vi "DriveFineAjust.vi"(8 "Fine Ajust F/B":dbl, 9 "Fine Ajust L/R":dbl, 10 "Right Side Normal":dbl, 11 "Left Side Normal":dbl) -> ()   [LabVIEW 2012]
uses:
  <vilib>/Rock Robotics/WPI/RobotDrive/WPI_RobotDriveGetSetRefNum.vi
  Max'sToolKit/ConvertVoltageToPercentVbs.vi
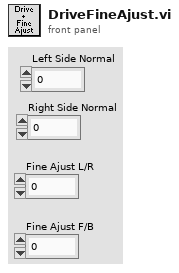
[diagram p1: front panel]
types:
  T1 = typedef "WPI_RobotDriveDevRef.ctl" = cluster{"DevStatus":errorcluster, "Motors[]":T2[], "Square Inputs":bool, "Max Output":dbl, "Isochronous":bool}
  T2 = typedef "WPI_MotorControlDeviceRef.ctl" = cluster{"DeviceStatus":errorcluster, "Type":enum16{"PWM", "CAN"}, "PWM":cluster{"Digital Module":T3, "PWM Channel":T4, "DeadBand":T5}, "CAN":cluster{"Device Number":u8, "Control Mode":T6, "Semaphore":T7, "Max Vout":dbl}, "Invert":bool, "TransformRef":T8, "InvTransformRef":T8}
  T3 = typedef "FPGA_TypedefDigitalModule.ctl" = enum16{"Digital Module 1", "Digital Module 2"}
  T4 = typedef "FPGA_DIOPWMChannel.ctl" = enum8{"PWM 1", "PWM 2", "PWM 3", "PWM 4", "PWM 5", "PWM 6", "PWM 7", "PWM 8", "PWM 9", "PWM 10", "Invalid"}
  T5 = typedef "WPI_PWMDeadband.ctl" = cluster{"Name":string, "maxPositivePwm":i32, "minPositivePwm":i32, "centerPwm":i32, "maxNegativePwm":i32, "minNegativePwm":i32, "angularRange":u16}
  T6 = typedef "WPI_CANJaguar_ControlMode.ctl" = enum8{"Percent VBus", "Current", "Speed", "Position", "Voltage"}
  T7 = typedef "Semaphore RefNum" = refnum<k1>
  T8 = typedef "WPI_PWMTransform_ConPane.ctl" = refnum<vi>
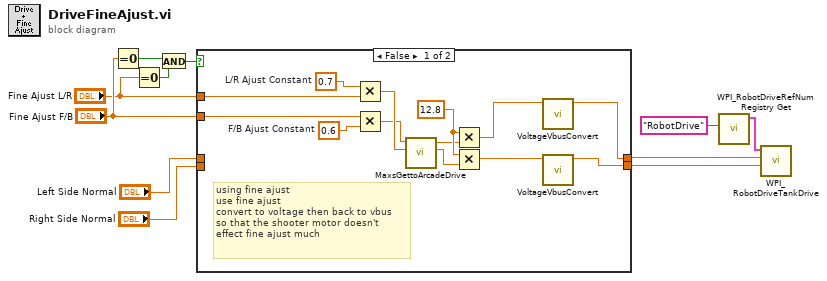
[diagram p0: block diagram]
diagram:
  n1 = Equal To 0?(x="Fine Ajust F/B") -> (x = 0?=w4:bool)
  n2 = Equal To 0?(x="Fine Ajust L/R") -> (x = 0?=w5:bool)
  n3 = And(x=w4, y=w5) -> (x .and. y?=w6:bool)
  n4 = case shown="False" w6 {
    tunnel: "Right Side Normal" -> [_ w25]
    tunnel: "Left Side Normal" -> [_ w26]
    tunnel: "Fine Ajust L/R" -> [w23 _]
    tunnel: "Fine Ajust F/B" -> [w21 _]
    tunnel: [w13 w26] -> w3
    tunnel: [w12 w25] -> w1
    frame False {
      w18 = 12.8
      w22 = 0.6  # F/B Ajust Constant
      w24 = 0.7  # L/R Ajust Constant
      # "using fine ajust\nuse fine ajust\nconvert to voltage then back to vbus\nso that the shooter motor doesn't\neffect fine ajust much"
      n5 = Multiply(x=w24, y=w23) -> (x*y=w20:dbl)
      n6 = Multiply(x=w21, y=w22) -> (x*y=w19:dbl)
      n7 = call "MaxsGettoArcadeDrive.vi"("Driver X In"=w20, "Driver Y In"=w19) -> ("Right Out"=w16:dbl, "Left Out"=w17:dbl)  [unwired: 8 in]
      n8 = Multiply(x=w18, y=w17) -> (x*y=w15:dbl)
      n9 = Multiply(x=w18, y=w16) -> (x*y=w14:dbl)
      n10 = call-poly "VoltageVbusConvert.vi"("Voltage"=w15) -> ("Vbus"=w13:dbl)  [unwired: 10 in]
      n11 = call-poly "VoltageVbusConvert.vi"("Voltage"=w14) -> ("Vbus"=w12:dbl)  [unwired: 10 in]
    }
    frame True {
      # "if neither fine ajust is being used then\nnormal tank drive"
    }
  }
  n12 = call <vilib>:"WPI_RobotDriveRefNum Registry Get.vi"("refnum name"="RobotDrive") -> ("RobotDriveDevRef"=w2:T1)  [unwired: 1 in, 9 out]
  n13 = call <vilib>:"WPI_RobotDriveTankDrive.vi"("Right axis value"=w1, "Left axis value"=w3, "RobotDriveDevRef"=w2) -> ()  [unwired: 6 in, 3 out]
